vi "Feather Size Read.vi"(4 "error in (no error)":errorcluster, 6 "Container State":T3, 7 "Display State In":T1) -> (0 "error out":errorcluster, 2 "Value":dbl, 3 "Display State Out":T1)   [LabVIEW 2017, in "2D Feather.xctl"]
uses:
  <vilib>/Math Plots/2D Math Plots/2D Feather/2D Feather XCtrl/2D Feather.xctl
  <vilib>/_xctls/Container State.ctl
  <vilib>/Math Plots/2D Math Plots/2D Feather/2D Feather XCtrl/State.ctl
  <vilib>/Math Plots/2D Math Plots/2D Feather/2D Feather/2D Feather.lvclass
  e:/builds/penguin/labview/branches/2017/dev/dist/vi.lib/Math Plots/2D Math Plots/2D Plot/2D Plot/2D Plot.lvclass
  <vilib>/Math Plots/2D Math Plots/2D Plot/Action String/2DMathPlot Ctrl Act Queue.ctl
  <vilib>/Math Plots/2D Math Plots/2D Plot/Action String/2DMathPlot Ctrl Act Cluster.ctl
  <vilib>/Math Plots/2D Math Plots/2D Plot/Action String/2DMathPlot State Class.ctl
  <vilib>/Math Plots/2D Math Plots/2D Plot/2D Plot/2D Plot.lvclass
  <vilib>/_xctls/XControlSupport.lvlib
panel:
  # "Replace the Value Indicator below with an Indicator of desired type.\nDo not remove this Indicator or the others from the connector pane. \nDo not change the connector pane pattern.\nThe Value Indicator should always be the second terminal from top on the output side in the connector pane."
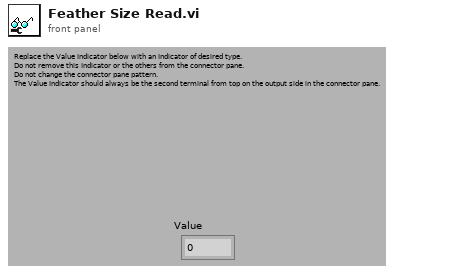
[diagram p1: front panel]
types:
  T1 = typedef "2D Feather.xctl/State.ctl" = cluster{"2D Feather.lvclass":refnum<class "2D Feather.lvclass">, "Control Ref Queue":T2, "Main Frame Color":u32, "Plot Legend Color":u32}
  T2 = typedef "2DMathPlot Ctrl Act Queue.ctl" = refnum<queue>
  T3 = typedef "XControlSupport.lvlib/Container State.ctl" = cluster{"Indicator?":bool, "Run Mode?":bool, " Refnum":refnum<vi>}
  T4 = typedef "2D Feather.lvclass/2D Feather Property Array.ctl" = T5[]
  T5 = typedef "2D Feather.lvclass/2D Feather Property.ctl" = cluster{"Arrow Size":dbl}
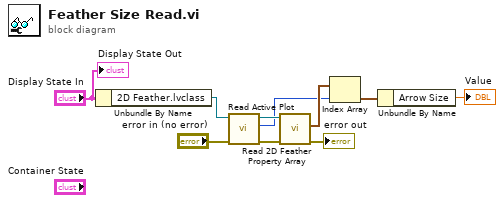
[diagram p0: block diagram]
diagram:
  n1 = Unbundle By Name("Display State In") -> ("2D Feather.lvclass"=w8:refnum<class "2D Feather.lvclass">)
  n2 = call <vilib>:"Read Active Plot.vi"("error in (no error)"="error in (no error)", "2D Plot.lvclass in"=w8) -> ("error out"=w5:errorcluster, "Active Plot"=w6:i32, "2D Plot.lvclass out"=w7:refnum<class "2D Feather.lvclass">)  [unwired: 7 out]
  n3 = call <vilib>:"Read 2D Feather Property Array.vi"("error in (no error)"=w5, "2D Feather.lvclass in"=w7) -> ("error out"=→"error out":errorcluster, "2D Feather Property Array"=w10:T4)  [unwired: 8 out]
  n4 = Index Array(array=w10, index=w6) -> (element=w9:T5)
  n5 = Unbundle By Name(w9) -> ("Arrow Size"=→"Value":dbl)
  "Display State Out" <- "Display State In"
